vi "Wiimote Enable Extension Controller.vi"(8 "error in":errorcluster, 11 "hWiimoteHandle in":u32 format="%08x") -> (0 "error out":errorcluster, 3 "hWiimoteHandle out":u32 format="%08x")   [LabVIEW 2010]
uses:
  Wiimote Address Space.ctl
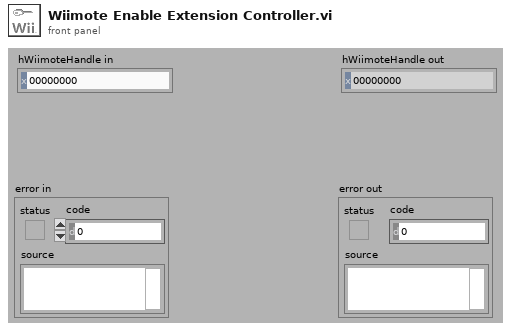
[diagram p1: front panel]
types:
  T1 = typedef "Wiimote Address Space.ctl" = u8
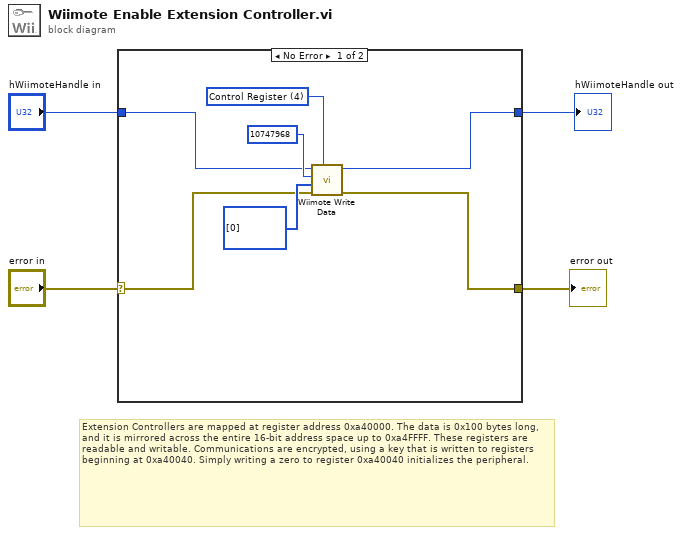
[diagram p0: block diagram]
diagram:
  # "Extension Controllers are mapped at register address 0xa40000. The data is 0x100 bytes long, and it is mirrored across the entire 16-bit address space up to 0xa4FFFF. These registers are readable and writable. Communications are encrypted, using a key that is written to registers beginning at 0xa40040. Simply writing a zero to register 0xa40040 initializes the peripheral."
  n1 = case shown="No Error" "error in" {
    selector: "error in" -> [w7 w13]
    tunnel: [w5 w13] -> w3
    tunnel: "hWiimoteHandle in" -> [w8 w12]
    tunnel: [w6 w12] -> w1
    frame No Error {
      w9 = T1 4 items=["EEPROM Memory"=0, "Control Register"=4] ("Address Space")
      n2 = call "Wiimote Write Data.vi"("Address Space"=w9, "error in"=w7, "pReportBuffer in"=u8[] [0], "Offset"=u32 10747968, "hWiimoteHandle in"=w8) -> ("error out"=w5:errorcluster, "hWiimoteHandle out"=w6:u32)  [unwired: 5 in]
    }
    frame Error {
    }
  }
  "error out" <- w3
  "hWiimoteHandle out" <- w1
